vi "EXCEL report.vi"(7 "Report state":T1=enum."Close report", 8 "error in":errorcluster, 10 "Data in":variant) -> (0 "error out":errorcluster, 2 "Data out":variant)   [LabVIEW 2016, in "Report.lvlib"]
uses:
  Report.lvlib
  TypeDefs/Report state.ctl
  TypeDefs/Report data.ctl
  <vilib>/Utility/NIReport.llb/NI_report.lvclass
  <vilib>/Utility/NIReport.llb/Append Numeric Table to Report (wrap).vi
  <vilib>/Utility/NIReport.llb/NI_ReportGenerationCore.lvlib
  <vilib>/Utility/NIReport.llb/Excel/NI_Excel.lvclass
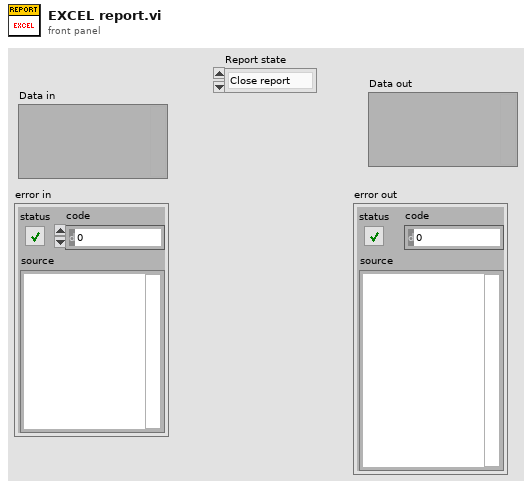
[diagram p1: front panel]
types:
  T1 = typedef "Report.lvlib/Report state.ctl" = enum16{"Create report", "Save data", "Save report", "Available printers", "Print report", "Close report"}
  T2 = enum16{"Standard Report", "HTML", "Word", "Excel"}
  T3 = enum16{"maximized", "minimized", "normal", "no change"}
  T4 = typedef "Report.lvlib/Report data.ctl" = cluster{"report ID":refnum<class "NI_report.lvclass">, "error":errorcluster}
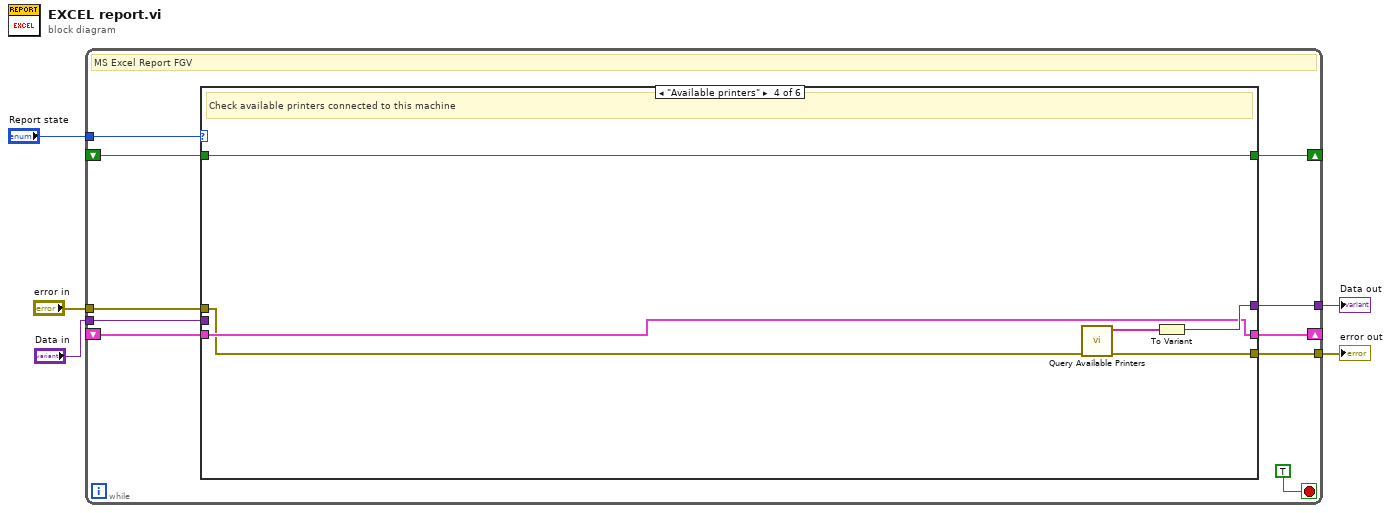
[diagram p0: block diagram]
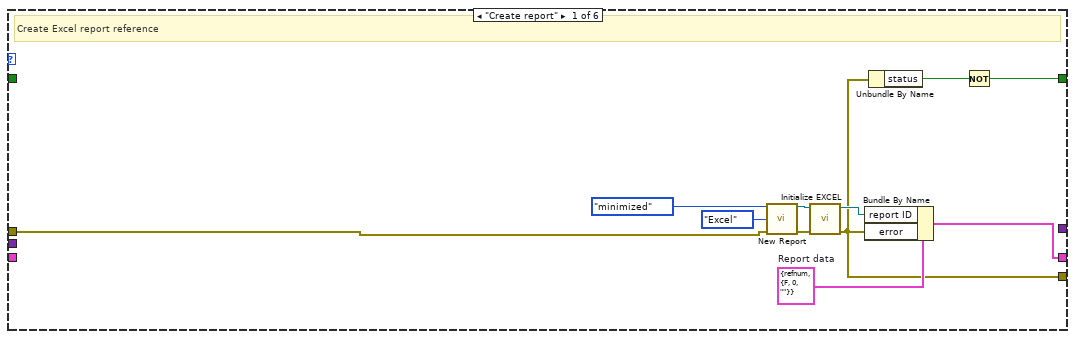
[diagram p2: hidden frame]
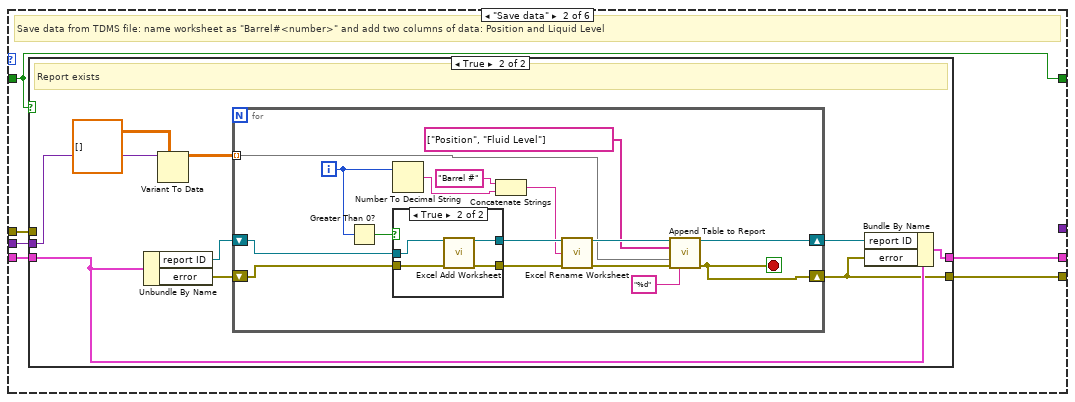
[diagram p3: hidden frame]
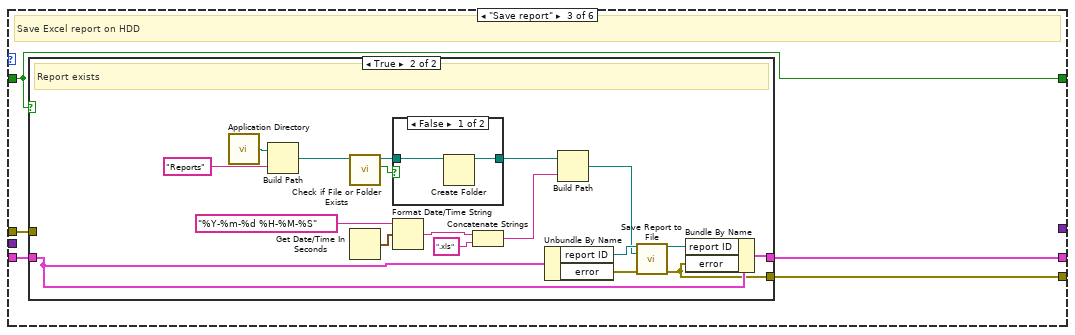
[diagram p6: hidden frame]
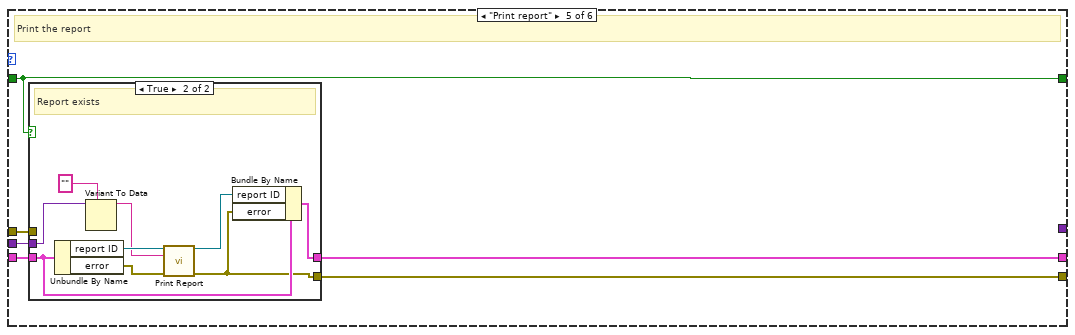
[diagram p9: hidden frame]
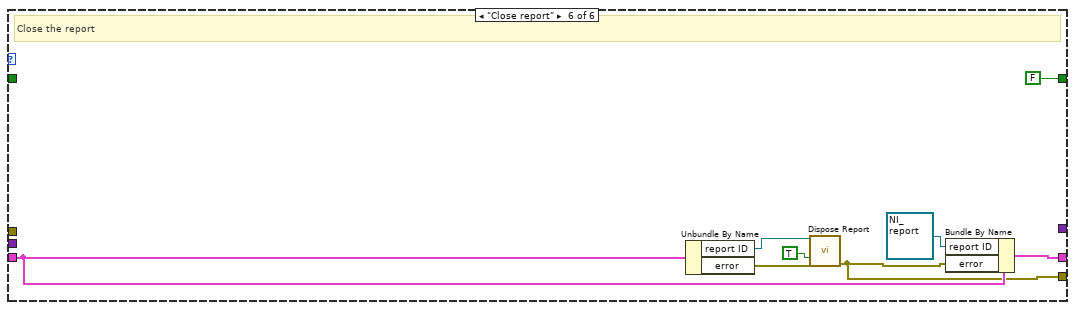
[diagram p11: hidden frame]
diagram:
  n1 = while {
    tunnel: "Report state" -> [w11]
    shift-right: [w13] -> _
    shift-left: _ -> [w14]
    tunnel: "Data in" -> [w12]
    tunnel: "error in" -> [w10]
    tunnel: [w9] -> w2
    tunnel: [w8] -> w1
    shift-right: [w6] -> _
    shift-left: _ -> [w7]
    stop <- TRUE stop-if-true
    # "MS Excel Report FGV"
    n2 = case shown="\"Available printers\"" w11 {
      tunnel: w14 -> [_ w32 w70 w97 w105 w123]
      tunnel: [w26 w31 w69 w97 w104 w124] -> w13
      tunnel: w12 -> [_ w30 _ _ w103 _]
      tunnel: w10 -> [w19 w27 w66 w96 w100 _]
      tunnel: [_ _ _ w98 _ _] -> w9
      tunnel: [w18 w29 w68 w95 w102 w118] -> w8
      tunnel: w7 -> [_ w28 w67 w94 w101 _]
      tunnel: [w16 w28 w67 w94 w101 FALSE] -> w6
      frame "Create report" {
        w20 = T4 {"report ID"=refnum, "error"={"status"=FALSE, "code"=0, "source"=""}}  # Report data
        # "Create Excel report reference"
        n3 = call <vilib>:"New Report.vi"("window state (normal)"=T3."minimized", "report type"=T2."Excel", "error in (no error)"=w19) -> ("report out"=w23:refnum<class "NI_report.lvclass">, "error out"=w22:errorcluster)  [unwired: 11 in]
        n4 = call "Initialize EXCEL.vi"("error in (no error)"=w22, "NI_report in"=w23) -> ("error out"=w18:errorcluster, "NI_report out"=w21:refnum<class "NI_report.lvclass">)  [unwired: 8 in]
        n5 = Bundle By Name(cluster=w20, "report ID"=w21, "error"=w18) -> (w26:T4)
        n6 = Unbundle By Name(w18) -> ("status"=w17:bool)
        n7 = Not(x=w17) -> (.not. x?=w16:bool)
      }
      frame "Save data" {
        # "Save data from TDMS file: name worksheet as \"Barrel#<number>\" and add two columns of data: Position and Liquid Level"
        n8 = case shown="True" w28 {
          tunnel: w32 -> [w33 w43]
          tunnel: [w33 w42] -> w31
          tunnel: w30 -> [_ w41]
          tunnel: [w34 w35] -> w29
          tunnel: w27 -> [w34 _]
          frame False {
            # "Report not created"
          }
          frame True {
            # "Report exists"
            n9 = Unbundle By Name(w43) -> ("report ID"=w37:refnum<class "NI_report.lvclass">, "error"=w40:errorcluster)
            n10 = Variant To Data(type=dbl[][][] [], Variant=w41) -> (data=w38:dbl[][][])  [unwired: 1 in, 1 out]
            n11 = for {
              tunnel: w38 -> [w48] mode=indexing
              shift-right: [w44] -> w35
              shift-left: w40 -> [w54]
              shift-right: [w49] -> w36
              shift-left: w37 -> [w55]
              i -> [w56]
              stop <- w44 stop-if-true
              n12 = Greater Than 0?(x=w56) -> (x > 0?=w57:bool)
              n13 = Number To Decimal String(number=w56) -> (decimal integer string=w58:string)  [unwired: 1 in]
              n14 = case shown="True" w57 {
                tunnel: w55 -> [w61 w65]
                tunnel: w54 -> [w60 w64]
                tunnel: [w61 w63] -> w53
                tunnel: [w60 w62] -> w52
                frame False {
                }
                frame True {
                  n15 = call <vilib>:"Excel Add Worksheet.vi"("report in"=w65, "error in (no error)"=w64) -> ("report out"=w63:refnum<class "NI_report.lvclass">, "error out"=w62:errorcluster)  [unwired: 12 in]
                }
              }
              n16 = Concatenate Strings("Barrel #", w58) -> (w47:string)
              n17 = call <vilib>:"Excel Rename Worksheet.vi"("report in"=w53, "worksheet name (\"\")"=w47, "error in (no error)"=w52) -> ("report out"=w51:refnum<class "NI_report.lvclass">, "error out"=w50:errorcluster)  [unwired: 11 in]
              n18 = call-poly <vilib>:"Append Table to Report.vi"("report in"=w51, "column headers"=string[] ["Position", "Fluid Level"], "numerical data"=w48, "error in (no error)"=w50, "format string (%.3f)"="%d") -> ("report out"=w49:refnum<class "NI_report.lvclass">, "error out"=w44:errorcluster)  [unwired: 7 in, 2 out]
            }
            n19 = Bundle By Name(cluster=w43, "report ID"=w36, "error"=w35) -> (w42:T4)
          }
        }
      }
      frame "Save report" {
        # "Save Excel report on HDD"
        n20 = case shown="True" w67 {
          tunnel: w70 -> [w71 w90]
          tunnel: [w71 w89] -> w69
          tunnel: [w72 w73] -> w68
          tunnel: w66 -> [w72 _]
          frame False {
            # "Report not created"
          }
          frame True {
            # "Report exists"
            n21 = call <vilib>:"Application Directory.vi"() -> ("Application Directory"=w79:path)
            n22 = Build Path(base path=w79, name or relative path="Reports") -> (appended path=w77:path)
            n23 = call <vilib>:"Check if File or Folder Exists.vi"("path"=w77) -> ("file or folder exists?"=w76:bool, "dup path"=w75:path)  [unwired: 8 in, 1 out]
            n24 = Get Date/Time In Seconds() -> (seconds since 1Jan1904=w84:timestamp)
            n25 = case shown="False" w76 {
              tunnel: w75 -> [w92 w93]
              tunnel: [w91 w93] -> w74
              frame False {
                n26 = Create Folder(path (use dialog)=w92) -> (created path=w91:path)  [unwired: 2 in, 2 out]
              }
              frame True {
              }
            }
            n27 = Format Date/Time String(time format string (%c)="%Y-%m-%d %H-%M-%S", seconds (now)=w84) -> (date/time string=w82:string)  [unwired: 1 in]
            n28 = Concatenate Strings(w82, ".xls" ("string")) -> (w80:string)
            n29 = Unbundle By Name(w90) -> ("report ID"=w88:refnum<class "NI_report.lvclass">, "error"=w87:errorcluster)
            n30 = Build Path(base path=w74, name or relative path=w80) -> (appended path=w85:path)
            n31 = call-dynamic "Save Report to File.vi"("report in"=w88, "report file path"=w85, "error in (no error)"=w87) -> ("report out"=w86:refnum<class "NI_report.lvclass">, "error out"=w73:errorcluster)  [unwired: 11 in]
            n32 = Bundle By Name(cluster=w90, "report ID"=w86, "error"=w73) -> (w89:T4)
          }
        }
      }
      frame "Available printers" {
        # "Check available printers connected to this machine"
        n33 = call <vilib>:"Query Available Printers.vi"("error in (no error)"=w96) -> ("error out"=w95:errorcluster, "system configured printers"=w99:string[])  [unwired: 8 in, 1 out]
        n34 = To Variant(anything=w99) -> (Variant=w98:variant)
      }
      frame "Print report" {
        # "Print the report"
        n35 = case shown="True" w101 {
          tunnel: w105 -> [w106 w114]
          tunnel: [w106 w113] -> w104
          tunnel: w103 -> [_ w111]
          tunnel: [w107 w108] -> w102
          tunnel: w100 -> [w107 _]
          frame False {
            # "Report not created"
          }
          frame True {
            # "Report exists"
            n36 = Unbundle By Name(w114) -> ("report ID"=w116:refnum<class "NI_report.lvclass">, "error"=w115:errorcluster)
            n37 = Variant To Data(type="", Variant=w111) -> (data=w109:string)  [unwired: 1 in, 1 out]
            n38 = call-dynamic "Print Report.vi"("report in"=w116, "printer name (default)"=w109, "error in (no error)"=w115) -> ("report out"=w112:refnum<class "NI_report.lvclass">, "error out"=w108:errorcluster)  [unwired: 11 in]
            n39 = Bundle By Name(cluster=w114, "report ID"=w112, "error"=w108) -> (w113:T4)
          }
        }
      }
      frame "Close report" {
        # "Close the report"
        n40 = Unbundle By Name(w123) -> ("report ID"=w122:refnum<class "NI_report.lvclass">, "error"=w121:errorcluster)
        n41 = call-dynamic "Dispose Report.vi"("report in"=w122, "save changes? (F)"=TRUE, "error in (no error)"=w121) -> ("error out"=w118:errorcluster)  [unwired: 12 in]
        n42 = Bundle By Name(cluster=w123, "report ID"=refnum<class "NI_report.lvclass"> refnum ("Report ID"), "error"=w118) -> (w124:T4)
      }
    }
  }
  "error out" <- w1
  "Data out" <- w2
